vi "11a-tmp.vi"() -> ()   [LabVIEW 2018]
panel:
  out "stopping":bool
  in  "stop polling 2":bool
  out "error out 2":errorcluster
  out "error out":errorcluster
  in  "stop polling":bool
  out "i":i32
  out "delay":i32
  out "Array":bool[](array[boolean])
  out "ixs":i32[](array[numeric])
  out "delays":i32[](array[numeric])
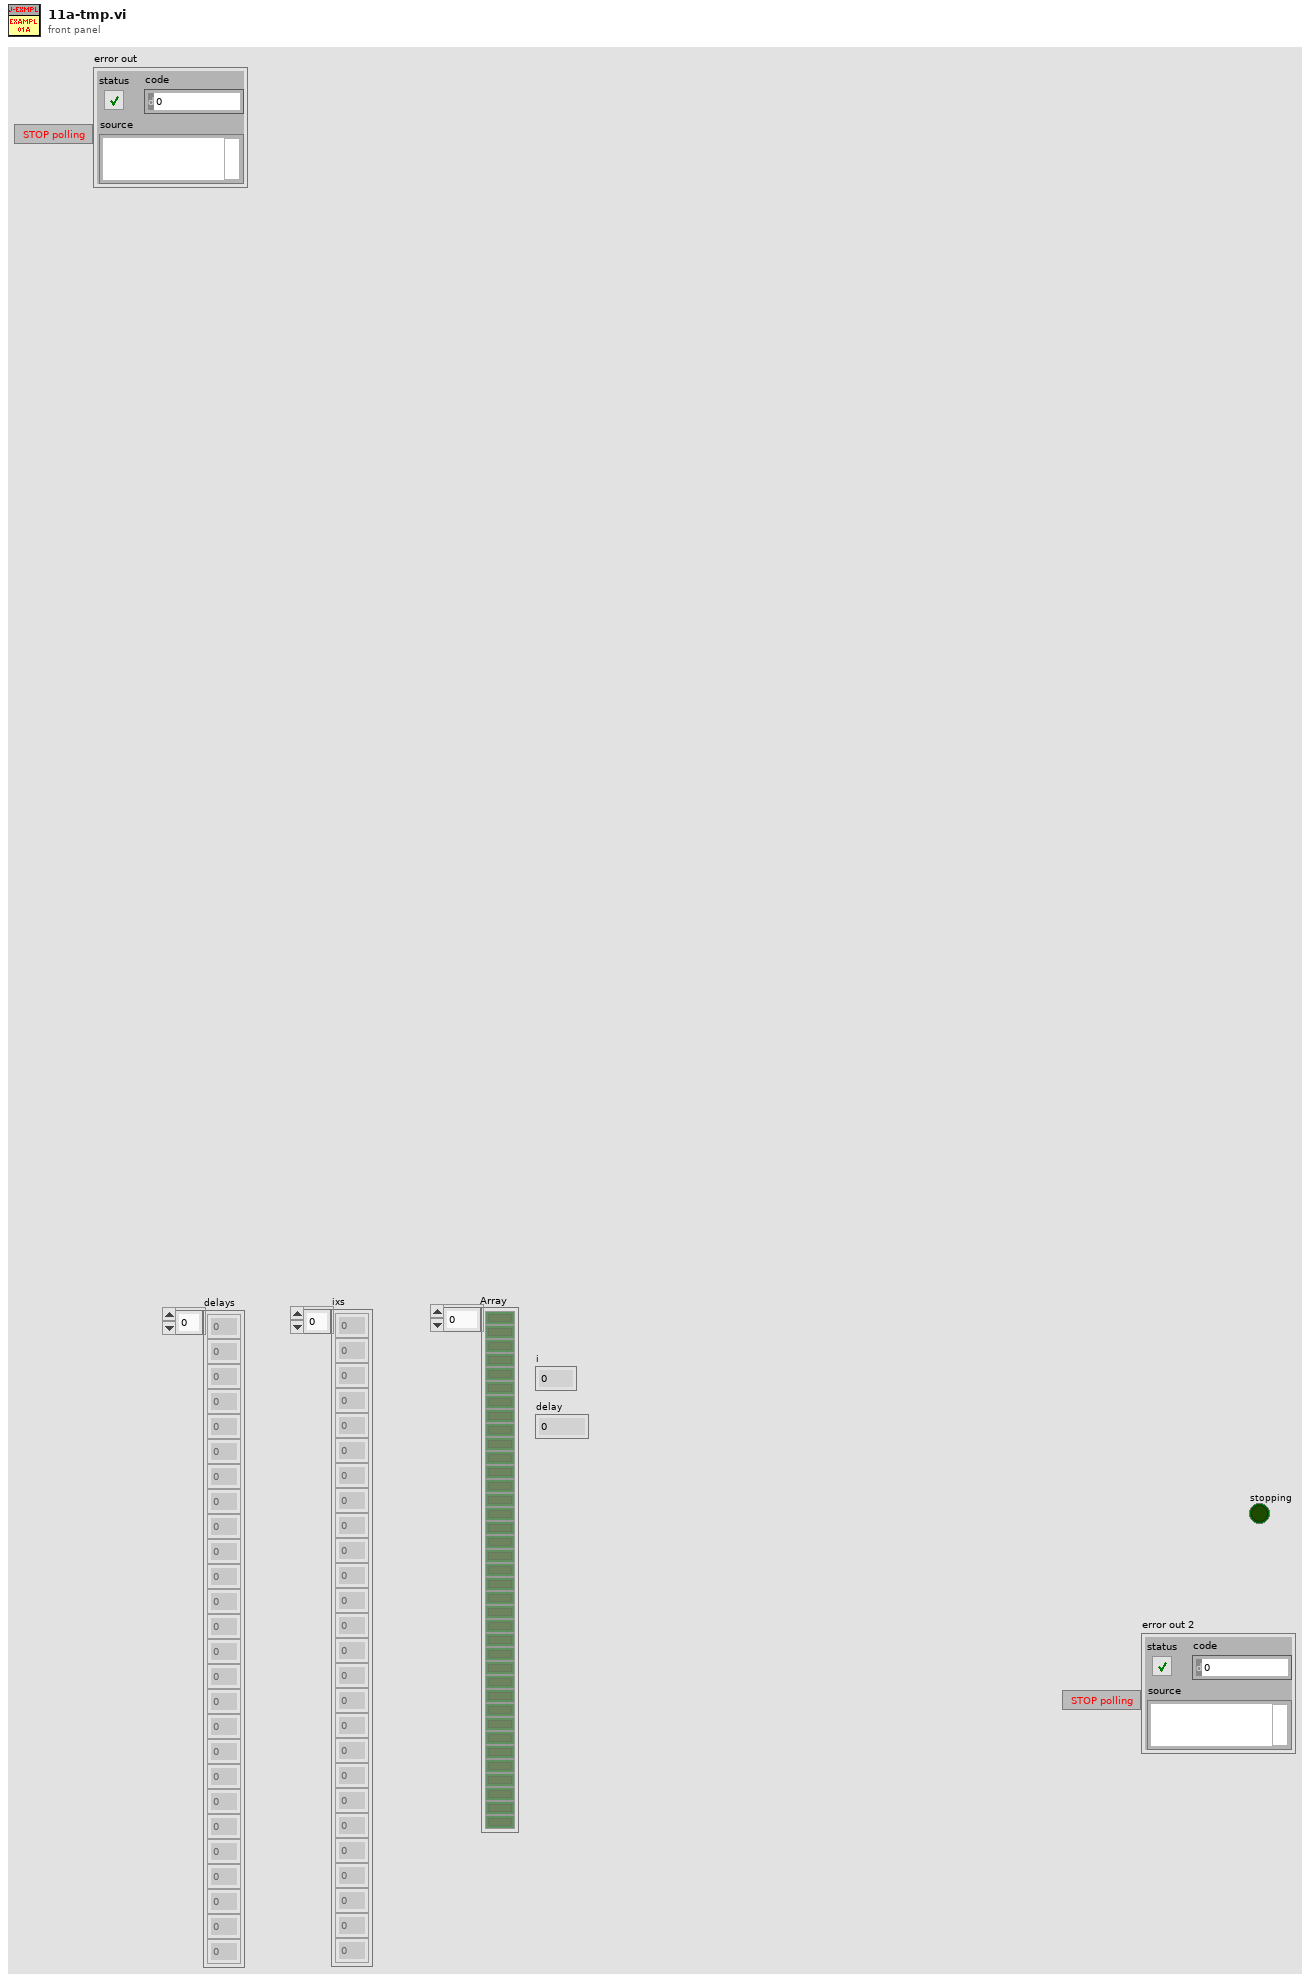
[diagram p1: front panel]
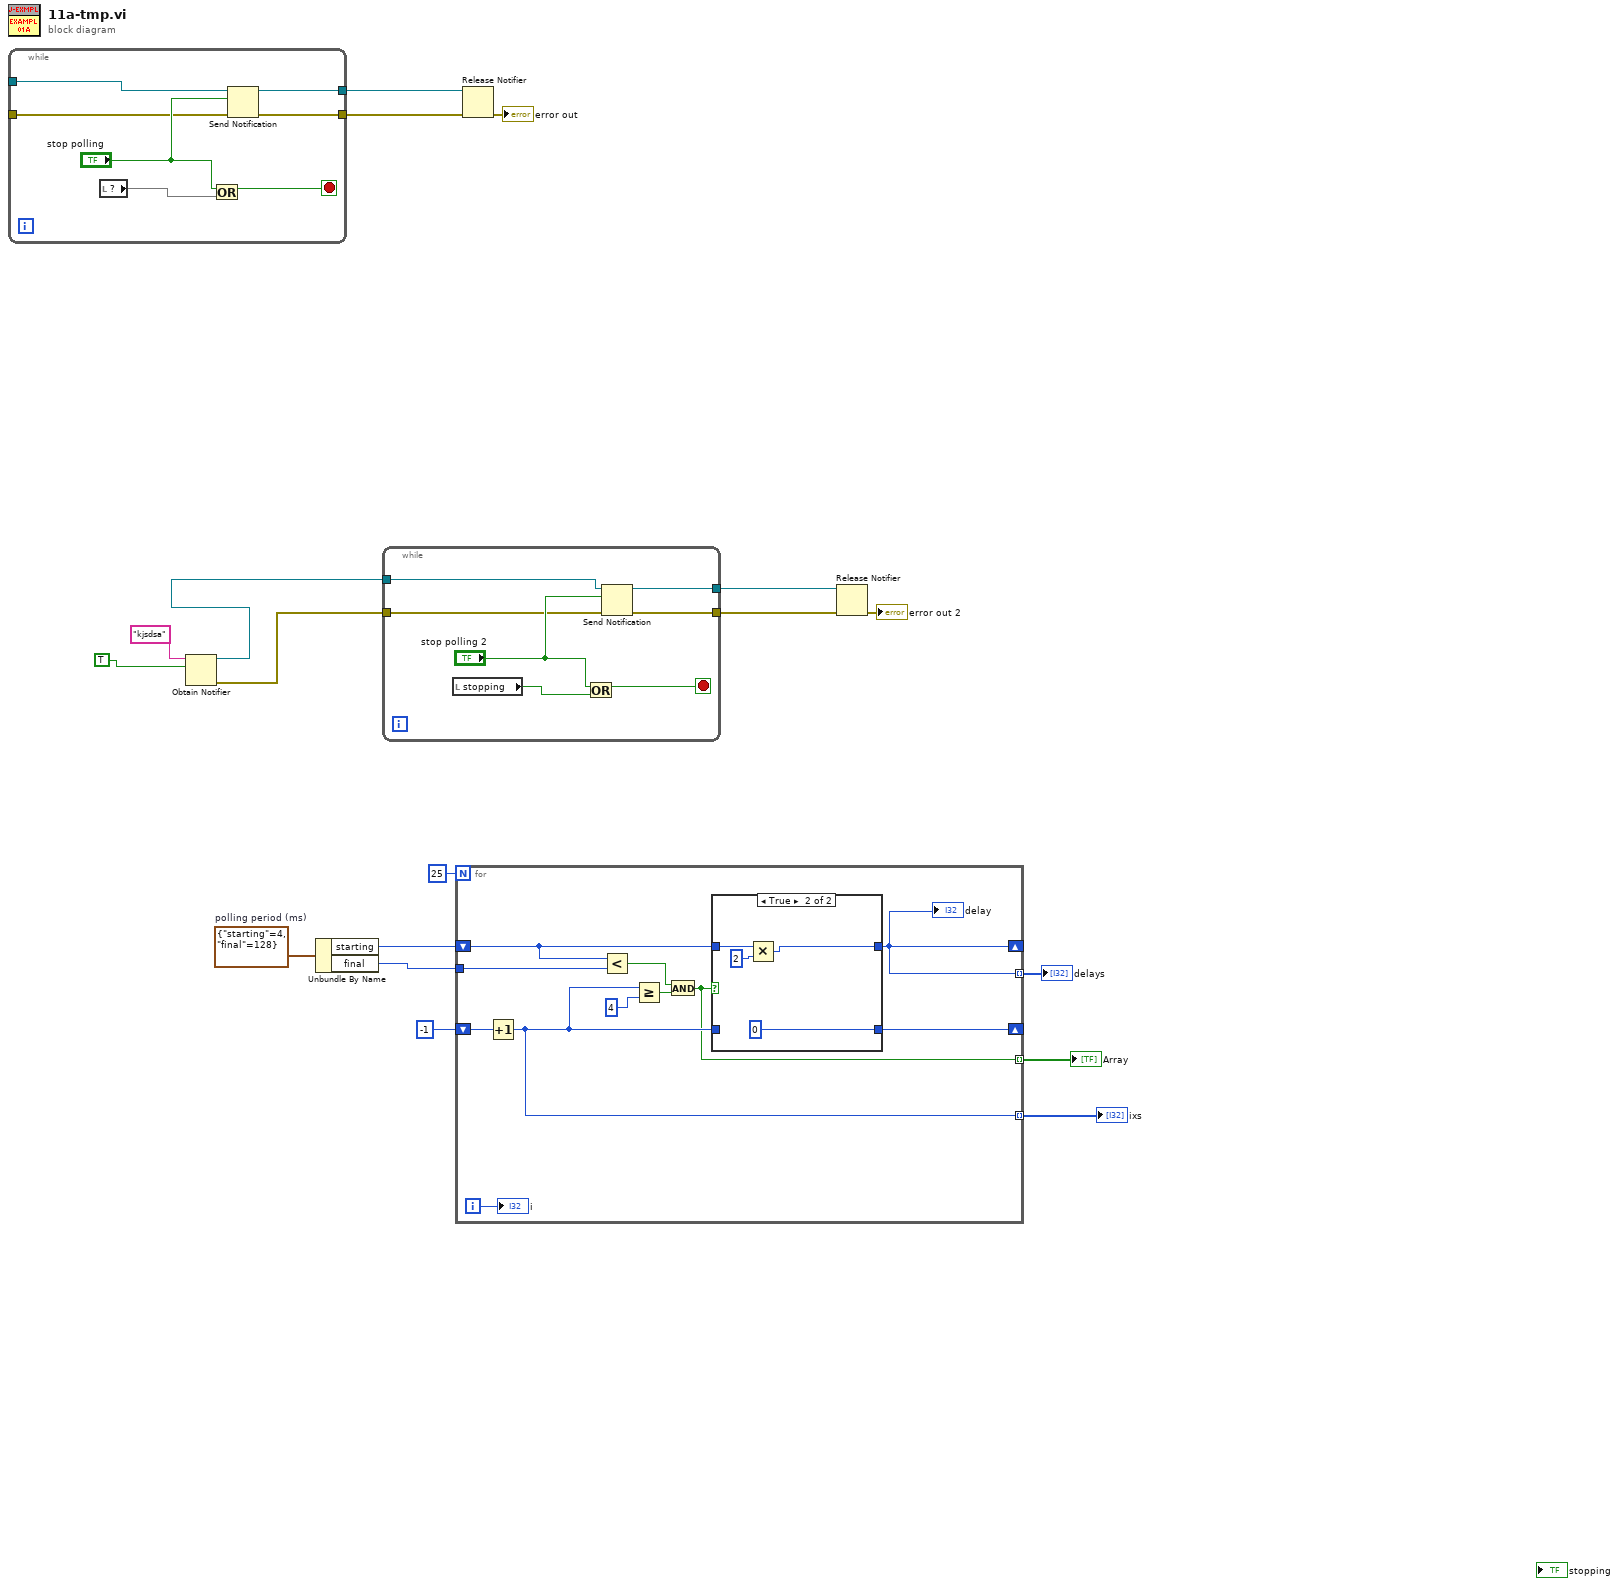
[diagram p0: block diagram]
diagram:
  w19 = cluster{"starting":i32, "final":i32} {"starting"=4, "final"=128}  # polling period (ms)
  n1 = while {
    tunnel: _ -> [w24]
    tunnel: [w22] -> w11
    tunnel: [w21] -> w10
    tunnel: [w20] -> w9
    stop <- w25 stop-if-true
    n2 = local read item#-1() -> (w26)
    n3 = Or(x="stop polling", y=w26) -> (x .or. y?=w25:bool)
    n4 = Send Notification(notification="stop polling", notifier=w24, error in (no error)=w21) -> (notifier out=w22:refnum<notifier>, error out=w20:errorcluster)
  }
  n5 = Obtain Notifier(name (unnamed)="kjsdsa", notification data type=TRUE) -> (notifier out=w3:refnum<notifier>, error out=w4:errorcluster)  [unwired: 2 in, 1 out]
  n6 = Unbundle By Name(w19) -> ("starting"=w18:i32, "final"=w16:i32)
  n7 = while {
    tunnel: w3 -> [w31]
    tunnel: [w29] -> w5
    tunnel: w4 -> [w28]
    tunnel: [w27] -> w6
    stop <- w32 stop-if-true
    n8 = local read "stopping"() -> (w33:bool)
    n9 = Or(x="stop polling 2", y=w33) -> (x .or. y?=w32:bool)
    n10 = Send Notification(notification="stop polling 2", notifier=w31, error in (no error)=w28) -> (notifier out=w29:refnum<notifier>, error out=w27:errorcluster)
  }
  n11 = for {
    N: 25 -> [_]
    shift-right: [w37] -> _
    shift-left: w18 -> [w38]
    shift-right: [w43] -> _
    shift-left: -1 ("counter") -> [w44]
    tunnel: w16 -> [w40]
    tunnel: [w37] -> w15 mode=indexing
    tunnel: [w36] -> w14 mode=indexing
    tunnel: [w35] -> w13 mode=indexing
    i -> [w34]
    n12 = Increment(x=w44) -> (x+1=w36:i32)
    n13 = Less?(x=w38, y=w40) -> (x < y?=w39:bool)
    n14 = Greater Or Equal?(x=w36, y=4) -> (x >= y?=w41:bool)
    n15 = And(x=w39, y=w41) -> (x .and. y?=w35:bool)
    n16 = case shown="True" w35 {
      tunnel: w36 -> [w46 _]
      tunnel: [w46 0] -> w43
      tunnel: w38 -> [w45 w49]
      tunnel: [w45 w48] -> w37
      frame False {
      }
      frame True {
        n17 = Multiply(x=w49, y=2) -> (x*y=w48:i32)
      }
    }
    "delay" <- w37
    "i" <- w34
  }
  "delays" <- w15
  "ixs" <- w14
  "Array" <- w13
  n18 = Release Notifier(notifier=w11, error in (no error)=w9) -> (error out=→"error out":errorcluster)  [unwired: 1 in, 2 out]
  n19 = Release Notifier(notifier=w5, error in (no error)=w6) -> (error out=→"error out 2":errorcluster)  [unwired: 1 in, 2 out]
